vi "Event handler-PMT value change.vi"   [LabVIEW 2017]
uses:
  Typedefs/PMT control functions.ctl
types:
  T1 = typedef "PMT control functions.ctl" = enum16{"Set PMTs from UI", "Reset PMTs"}
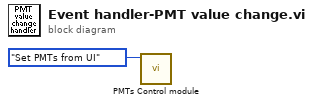
[diagram p0: block diagram]
diagram:
  n1 = call "PMTs Control module.vi"("Function"=PMT_control_functions."Set PMTs from UI") -> ()  [unwired: 10 in, 1 out]
